vi "Folder to first and last B Field.vi"(9 "B Field":i32, 10 "Wavenames":string[](array[string]), 11 "path":path) -> (2 "B Start":dbl, 3 "B Latest":dbl)   [LabVIEW 2016]
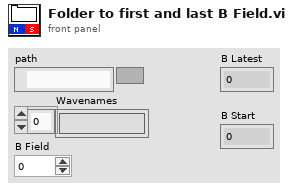
[diagram p1: front panel]
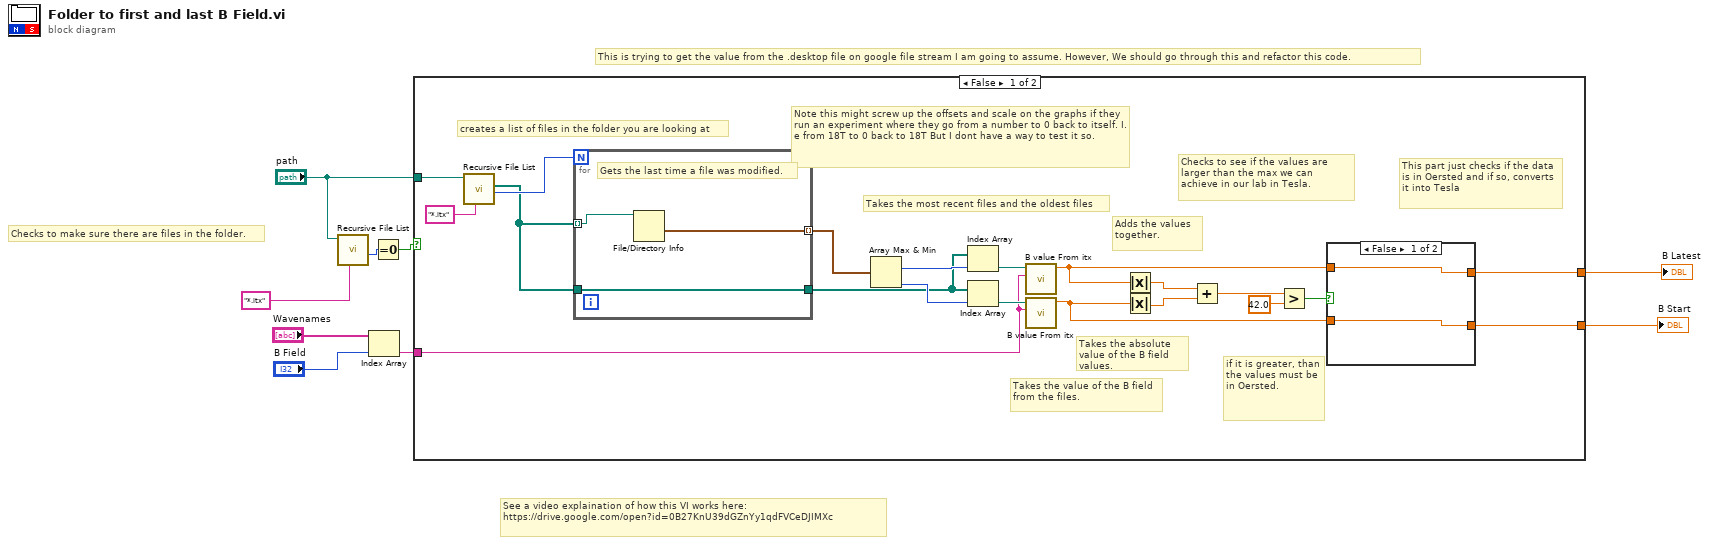
[diagram p0: block diagram]
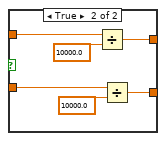
[diagram p2: hidden frame]
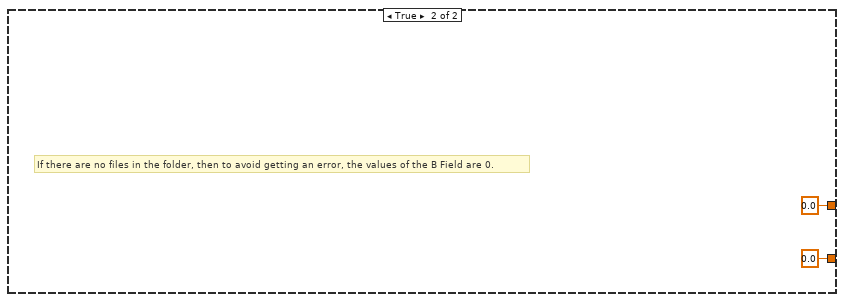
[diagram p3: hidden frame]
diagram:
  # "This is trying to get the value from the .desktop file on google file stream I am going to assume. However, We should go through this and refactor this code."
  # "Checks to make sure there are files in the folder."
  # "See a video explaination of how this VI works here: \nhttps://drive.google.com/open?id=0B27KnU39dGZnYy1qdFVCeDJIMXc"
  n1 = call <vilib>:"Recursive File List.vi"("pattern"="*.itx", "Folder Path"="path") -> ("Number of Files"=w6:i32)  [unwired: 5 in, 4 out]
  n2 = Index Array(array="Wavenames", index="B Field") -> (element=w2:string)
  n3 = Equal To 0?(x=w6) -> (x = 0?=w5:bool)
  n4 = case shown="False" w5 {
    tunnel: "path" -> [w23 _]
    tunnel: [w20 0.0 ("Numeric")] -> w9
    tunnel: [w19 0.0 ("Numeric")] -> w8
    tunnel: w2 -> [w11 _]
    frame False {
      # "if it is greater, than the values must be in Oersted."
      # "Checks to see if the values are larger than the max we can achieve in our lab in Tesla."
      # "Adds the values together."
      # "Takes the absolute value of the B field values."
      # "Takes the value of the B field from the files."
      # "Takes the most recent files and the oldest files"
      # "creates a list of files in the folder you are looking at"
      # "This part just checks if the data is in Oersted and if so, converts it into Tesla"
      # "Note this might screw up the offsets and scale on the graphs if they run an experiment where they go from a number to 0 back to itself. I.e from 18T to 0 back to 18T But I dont have a way to test it so."
      n5 = call <vilib>:"Recursive File List.vi"("pattern"="*.itx", "Folder Path"=w23) -> ("Number of Files"=w29:i32, "All Files in Dir"=w21:path[])  [unwired: 5 in, 3 out]
      n6 = for {
        N: w29 -> [_]
        tunnel: w21 -> [w39] mode=indexing
        tunnel: [w38] -> w24 mode=indexing
        tunnel: [w40] -> w22
        tunnel: w21 -> [w40]
        # "Gets the last time a file was modified."
        n7 = File/Directory Info(path=w39) -> (last mod=w38:timestamp)  [unwired: 1 in, 6 out]
      }
      n8 = Array Max & Min(array=w24) -> (max index (indices)=w25:i32, min index (indices)=w28:i32)  [unwired: 2 out]
      n9 = Index Array(array=w22, index=w25) -> (element=w27:path)
      n10 = Index Array(array=w22, index=w28) -> (element=w26:path)
      n11 = call "B value From itx.vi"("B Field Name"=w11, "file (use dialog)"=w27) -> ("Numeric"=w13:dbl)  [unwired: 9 in]
      n12 = call "B value From itx.vi"("B Field Name"=w11, "file (use dialog)"=w26) -> ("Numeric"=w12:dbl)  [unwired: 9 in]
      n13 = Absolute Value(x=w13) -> (abs(x)=w18:dbl)
      n14 = Absolute Value(x=w12) -> (abs(x)=w17:dbl)
      n15 = Add(x=w18, y=w17) -> (x+y=w16:dbl)
      n16 = Greater?(x=w16, y=42.0) -> (0:w14:bool)
      n17 = case shown="False" w14 {
        tunnel: w12 -> [w30 w37]
        tunnel: [w31 w36] -> w20
        tunnel: [w30 w35] -> w19
        tunnel: w13 -> [w31 w32]
        frame False {
        }
        frame True {
          n18 = Divide(x=w32, y=10000.0) -> (x/y=w36:dbl)
          n19 = Divide(x=w37, y=10000.0) -> (x/y=w35:dbl)
        }
      }
    }
    frame True {
      # "If there are no files in the folder, then to avoid getting an error, the values of the B Field are 0."
    }
  }
  "B Latest" <- w9
  "B Start" <- w8
